vi "Write Value.vi"(8 "error in (no error)":errorcluster, 10 "Value":path, 11 "Boolean Parameter in":refnum<class "File Path Parameter.lvclass">) -> (0 "error out":errorcluster, 3 "Boolean Parameter out":refnum<class "File Path Parameter.lvclass">)   [LabVIEW 2016, in "CD Parameter Manager API.lvlib" / "File Path Parameter.lvclass"]
uses:
  File Path Parameter.lvclass
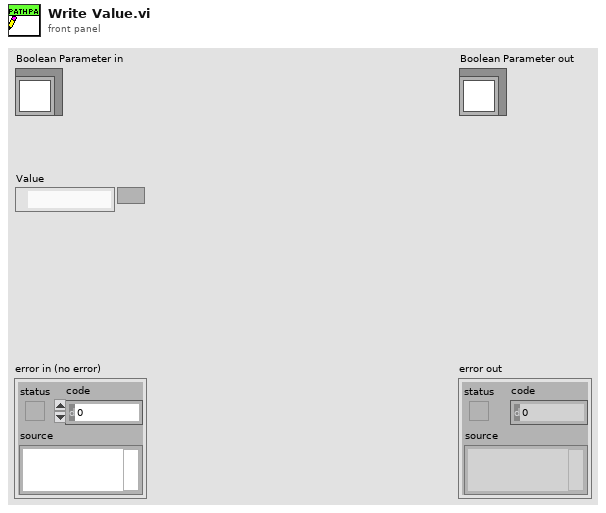
[diagram p1: front panel]
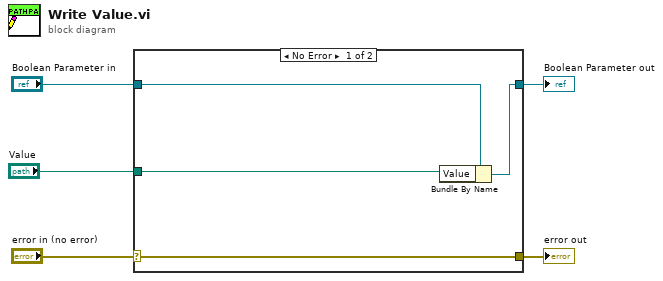
[diagram p0: block diagram]
diagram:
  n1 = case shown="No Error" "error in (no error)" {
    selector: "error in (no error)" -> [w9 w10]
    tunnel: [w9 w10] -> w4
    tunnel: [w7 w11] -> w2
    tunnel: "Boolean Parameter in" -> [w8 w11]
    tunnel: "Value" -> [w6 _]
    frame No Error {
      n2 = Bundle By Name(cluster=w8, "Value"=w6) -> (w7:refnum<class "File Path Parameter.lvclass">)
    }
    frame Error {
    }
  }
  "error out" <- w4
  "Boolean Parameter out" <- w2
